vi "Op-Stress-Status.vi"(8 "error in (no error)":errorcluster, 9 "operation":bool, 11 "VISA session":refnum<visa-resource-name>) -> (0 "error out":errorcluster, 1 "rate (%)":dbl format="%^.6e", 2 "time (sec)":dbl format="%^.6e", 3 "VISA resource name out":refnum<visa-resource-name>)   [LabVIEW 2016, in "Agilent 415X Series.lvlib"]
doc: "This VI monitors or resets the stress status value."
uses:
  Agilent 415X Series.lvlib
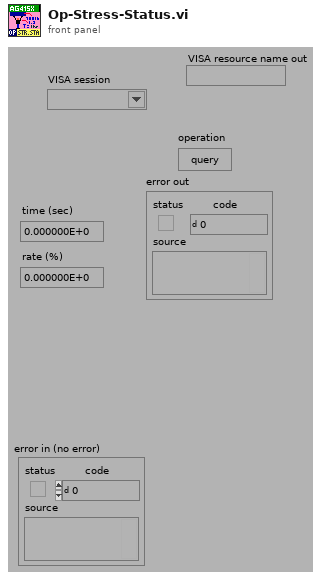
[diagram p1: front panel]
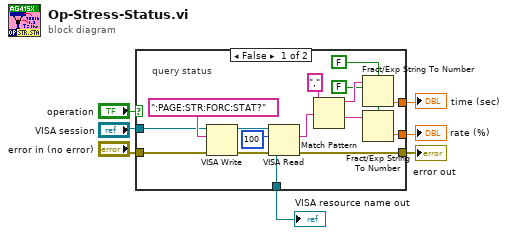
[diagram p0: block diagram]
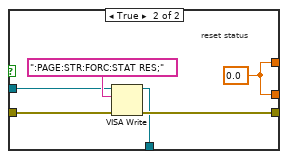
[diagram p2: hidden frame]
diagram:
  n1 = case shown="False" "operation" {
    tunnel: "error in (no error)" -> [w20 w28]
    tunnel: "VISA session" -> [w19 w27]
    tunnel: [w14 w26] -> w3
    tunnel: [w13 w26] -> w2
    tunnel: [w12 w25] -> w4
    tunnel: [w8 w24] -> w1
    frame False {
      # "query status"
      n2 = VISA Write(VISA resource name=w19, write buffer=":PAGE:STR:FORC:STAT?", error in (no error)=w20) -> (VISA resource name out=w22:refnum<visa-resource-name>, error out=w23:errorcluster)  [unwired: 1 out]
      n3 = VISA Read(VISA resource name=w22, byte count=u32 100, error in (no error)=w23) -> (VISA resource name out=w8:refnum<visa-resource-name>, read buffer=w18:string, error out=w12:errorcluster)  [unwired: 1 out]
      n4 = Match Pattern(string=w18, regular expression=",") -> (before substring=w15:string, after substring=w16:string)  [unwired: 1 in, 2 out]
      n5 = Fract/Exp String To Number(use system decimal point (T)=FALSE, string=w15) -> (number=w14:dbl)  [unwired: 2 in, 1 out]
      n6 = Fract/Exp String To Number(use system decimal point (T)=FALSE, string=w16) -> (number=w13:dbl)  [unwired: 2 in, 1 out]
    }
    frame True {
      w26 = 0.0
      # "reset status"
      n7 = VISA Write(VISA resource name=w27, write buffer=":PAGE:STR:FORC:STAT RES;", error in (no error)=w28) -> (VISA resource name out=w24:refnum<visa-resource-name>, error out=w25:errorcluster)  [unwired: 1 out]
    }
  }
  "time (sec)" <- w3
  "error out" <- w4
  "rate (%)" <- w2
  "VISA resource name out" <- w1
